vi "SVXMPL_Convert Wav to WDT.vi"(4 "stereo 16-bit":i16[][](array[numeric]), 5 "mono 16-bit":i16[](array[numeric]), 6 "stereo 8-bit":u8[][](array[numeric]), 7 "mono 8-bit":u8[](array[numeric]), 8 "error in (no error)":errorcluster, 10 "sound format":T1={"sound quality"=enum."mono", "rate"=enum."44100", "bits per sample"=enum."16 bit"}, 11 "Gain":dbl=1.0 format="%.2f") -> (0 "error out":errorcluster, 2 "Channel 2":waveform(dbl), 3 "Channel 1":waveform(dbl))   [LabVIEW 2017]
uses:
  <vilib>/sound/lvsound.llb/Sound Format.ctl
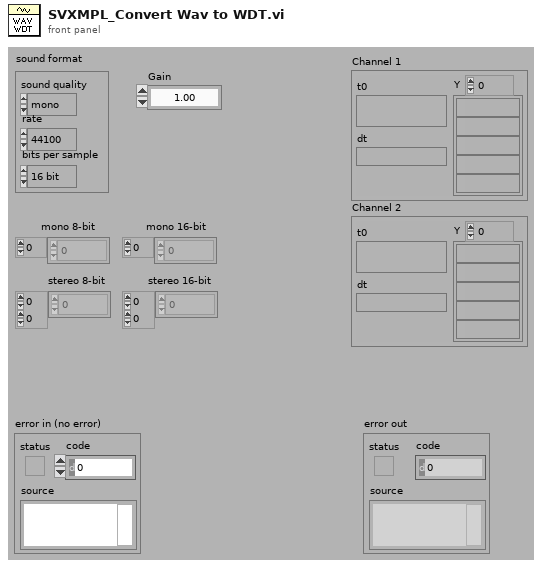
[diagram p1: front panel]
types:
  T1 = typedef "Sound Format.ctl" = cluster{"sound quality":enum16{"mono", "stereo"}, "rate":enum16{"11025", "22050", "44100", "8000"}, "bits per sample":enum16{"8 bit", "16 bit"}}
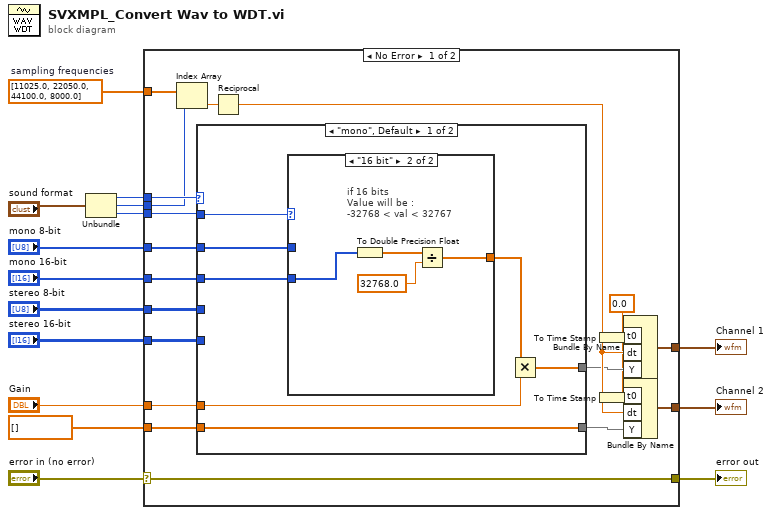
[diagram p0: block diagram]
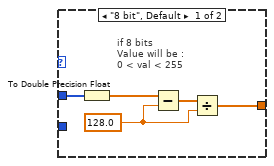
[diagram p2: hidden frame]
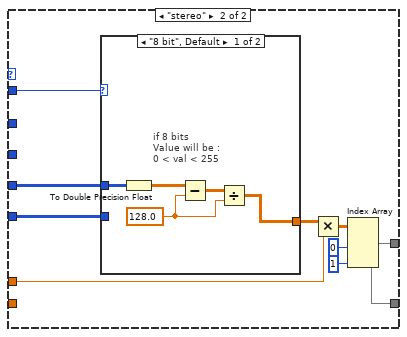
[diagram p3: hidden frame]
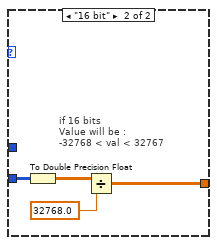
[diagram p4: hidden frame]
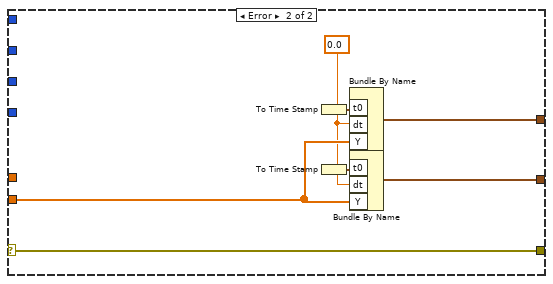
[diagram p5: hidden frame]
diagram:
  w6 = dbl[] [11025.0, 22050.0, 44100.0, 8000.0]  # sampling frequencies
  n1 = Unbundle("sound format") -> ("sound quality"=w10:enum16{"mono", "stereo"}, "rate"=w7:enum16{"11025", "22050", "44100", "8000"}, "bits per sample"=w13:enum16{"8 bit", "16 bit"})
  n2 = case shown="No Error" "error in (no error)" {
    selector: "error in (no error)" -> [w19 w77]
    tunnel: [w19 w77] -> w11
    tunnel: w10 -> [w35 _]
    tunnel: w13 -> [w34 _]
    tunnel: "mono 8-bit" -> [w33 _]
    tunnel: "mono 16-bit" -> [w32 _]
    tunnel: "Gain" -> [w31 _]
    tunnel: w7 -> [w29 _]
    tunnel: w6 -> [w28 _]
    tunnel: "stereo 8-bit" -> [w27 _]
    tunnel: "stereo 16-bit" -> [w26 _]
    tunnel: [w21 w76] -> w3
    tunnel: [w20 w75] -> w2
    tunnel: dbl[] [] -> [w18 w74]
    frame No Error {
      w22 = 0.0 ("t0")
      n3 = Index Array(array=w28, index=w29) -> (element=w30:dbl)
      n4 = case shown="\"mono\", Default" w35 {
        tunnel: w34 -> [w42 w61]
        tunnel: w33 -> [w41 _]
        tunnel: w32 -> [w40 _]
        tunnel: w31 -> [w38 w58]
        tunnel: w27 -> [_ w60]
        tunnel: w26 -> [_ w56]
        tunnel: [w37 w55] -> w24
        tunnel: [w36 w54] -> w23
        tunnel: w18 -> [w36 _]
        frame "mono", Default {
          n5 = case shown="\"16 bit\"" w42 {
            tunnel: w40 -> [_ w51]
            tunnel: w41 -> [w45 _]
            tunnel: [w46 w49] -> w39
            frame "8 bit", Default {
              w43 = 128.0 ("ratio")
              # "if 8 bits\nValue will be :\n0 < val < 255"
              n6 = To Double Precision Float(number=w45) -> (double precision float=w44:dbl[])
              n7 = Subtract(x=w44, y=w43) -> (x-y=w47:dbl[])
              n8 = Divide(x=w47, y=w43) -> (x/y=w46:dbl[])
            }
            frame "16 bit" {
              # "if 16 bits\nValue will be :\n-32768 < val < 32767"
              n9 = To Double Precision Float(number=w51) -> (double precision float=w48:dbl[])
              n10 = Divide(x=w48, y=32768.0 ("ratio")) -> (x/y=w49:dbl[])
            }
          }
          n11 = Multiply(x=w39, y=w38) -> (x*y=w37:dbl[])
        }
        frame "stereo" {
          n12 = case shown="\"8 bit\", Default" w61 {
            tunnel: w60 -> [w63 _]
            tunnel: [w62 w67] -> w59
            tunnel: w56 -> [_ w68]
            frame "8 bit", Default {
              w64 = 128.0 ("ratio")
              # "if 8 bits\nValue will be :\n0 < val < 255"
              n13 = To Double Precision Float(number=w63) -> (double precision float=w65:dbl[][])
              n14 = Subtract(x=w65, y=w64) -> (x-y=w66:dbl[][])
              n15 = Divide(x=w66, y=w64) -> (x/y=w62:dbl[][])
            }
            frame "16 bit" {
              # "if 16 bits\nValue will be :\n-32768 < val < 32767"
              n16 = To Double Precision Float(number=w68) -> (double precision float=w69:dbl[][])
              n17 = Divide(x=w69, y=32768.0 ("ratio")) -> (x/y=w67:dbl[][])
            }
          }
          n18 = Multiply(x=w59, y=w58) -> (x*y=w57:dbl[][])
          n19 = Index Array(array=w57, index (col) #1=0 ("Disabled Index (col)"), index (col) #2=1 ("Index (col)")) -> (element #1=w55:dbl[], element #2=w54:dbl[])  [unwired: 2 in]
        }
      }
      n20 = Reciprocal(x=w30) -> (1/x=w25:dbl)
      n21 = To Time Stamp(1:w22) -> (0:w16:timestamp)
      n22 = To Time Stamp(1:w22) -> (0:w17:timestamp)
      n23 = Bundle By Name("t0"=w16, "dt"=w25, "Y"=w24) -> (w21:waveform(dbl))  [unwired: 1 in]
      n24 = Bundle By Name("t0"=w17, "dt"=w25, "Y"=w23) -> (w20:waveform(dbl))  [unwired: 1 in]
    }
    frame Error {
      w73 = 0.0 ("t0")
      n25 = To Time Stamp(1:w73) -> (0:w71:timestamp)
      n26 = To Time Stamp(1:w73) -> (0:w72:timestamp)
      n27 = Bundle By Name("t0"=w71, "dt"=w73, "Y"=w74) -> (w76:waveform(dbl))  [unwired: 1 in]
      n28 = Bundle By Name("t0"=w72, "dt"=w73, "Y"=w74) -> (w75:waveform(dbl))  [unwired: 1 in]
    }
  }
  "error out" <- w11
  "Channel 1" <- w3
  "Channel 2" <- w2
